vi "Close.vi"(8 "error in (no error)":errorcluster, 11 "Menu in":refnum<class "Menu.lvclass">) -> (0 "error out":errorcluster)   [LabVIEW 2021, in "Menu.lvlib" / "Menu.lvclass"]
uses:
  Menu.lvclass
  TD_CloseEvent.ctl
  <vilib>/event_ctls.llb/usereventprio.ctl
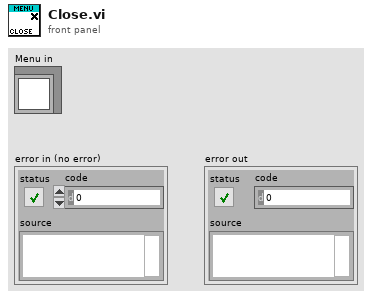
[diagram p1: front panel]
types:
  T1 = typedef "usereventprio.ctl" = enum32{"high priority", "normal priority"}
  T2 = typedef "Menu.lvlib/Menu.lvclass/TD_CloseEvent.ctl" = cluster{"Close":bool}
  T3 = typedef "Menu.lvlib/Menu.lvclass/Data.ctl" = cluster{"MenuMap":map{string, T4}, "PictRef":refnum<vi>, "MenuSelectionEvent":refnum<user-event>, "TopMenuSpacing":i32, "MenuSpacing":i32, "CloseEvent":refnum<user-event>, "TR_ManageMenuRef":refnum<vi>, "MenuColors":T6, "RTMPath":path, "RTMVIReference":refnum<vi>, "RTMMenuReference":refnum<k9>, "CtlRef":refnum<vi>, "User-Specified Font":refnum<class "Font.lvclass">, "Desired Font":enum16{"User-specified Font", "Application Font", "System Font", "Dialog Font"}, "SubMenuIcon":T7, "SubMenuIconClosed":refnum<class "Picture2D.lvclass">, "SubMenuIconOpened":refnum<class "Picture2D.lvclass">}
  T4 = typedef "Menu.lvlib/Menu.lvclass/MenuItems.ctl" = cluster{"Item Name":string, "Short Cut":T5, "Checked":bool, "Enable":bool, "After item":string, "Item Tags":string[], "Item Names":string[], "Picture":refnum<class "Image.lvclass">, "Hilite Picture":refnum<class "Image.lvclass">, "Displayed":bool}
  T5 = typedef "LVMenuShortCut.ctl" = cluster{"Include Shift Key?":bool, "Include Ctrl Key?":bool, "Shortcut Key":string}
  T6 = typedef "Menu.lvlib/Menu.lvclass/MenuColors.ctl" = cluster{"Text":refnum<class "Color.lvclass">, "HiliteText":refnum<class "Color.lvclass">, "Background":refnum<class "Color.lvclass">, "BorderColor":refnum<class "Color.lvclass">, "Hilite":refnum<class "Color.lvclass">}
  T7 = typedef "Menu.lvlib/Menu.lvclass/SubMenuIcon.ctl" = enum16{"LabVIEW", "Windows", "Custom"}
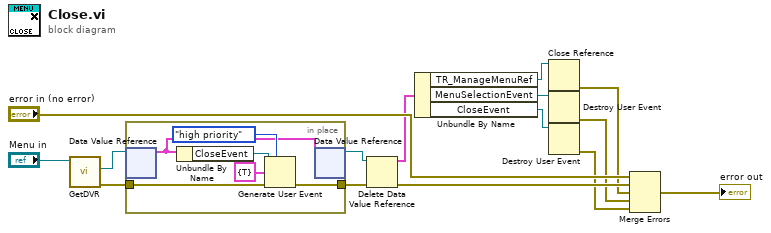
[diagram p0: block diagram]
diagram:
  n1 = call "GetDVR.vi"("Menu in"="Menu in") -> ("error out"=w6:errorcluster, "DVR"=w3:refnum<data-value>)  [unwired: 8 in, 1 out]
  n2 = in-place {
    in-place-border: [w20] -> w5
    in-place-border: w6 -> [w21]
    n3 = in-place-dvr #1(w3) -> (w16:T3)  [unwired: 1 out]
    n4 = Unbundle By Name(w16) -> ("CloseEvent"=w19:refnum<user-event>)
    n5 = Generate User Event(priority (normal)=usereventprio."high priority", user event=w19, event data cluster=T2 {"Close"=TRUE} ("event data"), error in=w21) -> (error out=w20:errorcluster)  [unwired: 1 out]
    n6 = in-place-dvr #1(w16) -> (w4:refnum<data-value>)  [unwired: 1 out]
  }
  n7 = Delete Data Value Reference(data value reference=w4, error in=w5) -> (data value=w11:T3, error out=w12:errorcluster)
  n8 = Unbundle By Name(w11) -> ("TR_ManageMenuRef"=w2:refnum<vi>, "MenuSelectionEvent"=w10:refnum<user-event>, "CloseEvent"=w9:refnum<user-event>)
  n9 = Close Reference(reference=w2) -> (error out=w1:errorcluster)  [unwired: 1 in]
  n10 = Destroy User Event(user event=w10) -> (error out=w7:errorcluster)  [unwired: 1 in]
  n11 = Destroy User Event(user event=w9) -> (error out=w8:errorcluster)  [unwired: 1 in]
  n12 = Merge Errors("error in (no error)", w12, w1, w7, w8) -> (→"error out":errorcluster)
